vi "5800PRStatus.vi"(6 "VISA resource name":refnum<visa-resource-name>="GPIB::1") -> (9 "Gain":u16(ring) items=["20.0 dB", "40.0 dB", "60.0 dB"], 10 "Pan Scan Settings":T1, 11 "no 5800?":bool, 12 "Operation Mode":u16(ring) items=["Pulse-Echo", "Through", "External Pulser"], 13 "Output Attenuation":dbl=5.0 format="%.1g", 14 "Pulser Repitition Frequency":u16(ring)=10 items=["External Remote", "External BNC", "0.080 KHz", "0.100 KHz", "0.125 KHz", "0.160 KHz", "0.200 KHz", "0.250 KHz", "0.400 KHz", "0.500 KHz", "1.000 KHz", "1.250 KHz", "2.000 KHz", "2.500 KHz", "4.000 KHz", "5.000 KHz", "10.000 KHz"], 15 "Energy Level":u16(ring)=1 items=["12.5 uJ", "25.0 uJ", "50.0 uJ", "100.0 uJ"], 16 "Damping Value":u16(ring)=3 items=["15 ohms", "17 ohms", "21 ohms", "25 ohms", "36 ohms", "50 ohms", "100 ohms", "500 ohms"], 17 "Highpass Filter Frequency":u16(ring) items=["1 KHz", "100 KHz", "300 KHz", "1000 KHz"], 18 "Lowpass Filter Frequency":u16(ring)=3 items=["5 MHz", "10 MHz", "20 MHz", "35 MHz"], 19 "Input Attenuation":u16(ring)=1 items=["0.0 dB", "10.0 dB", "20.0 dB", "30.0 dB", "40.0 dB", "50.0 dB"])   [LabVIEW 2022 SP3]
panel:
  # "This VI returns the present setting of the 5800PR"
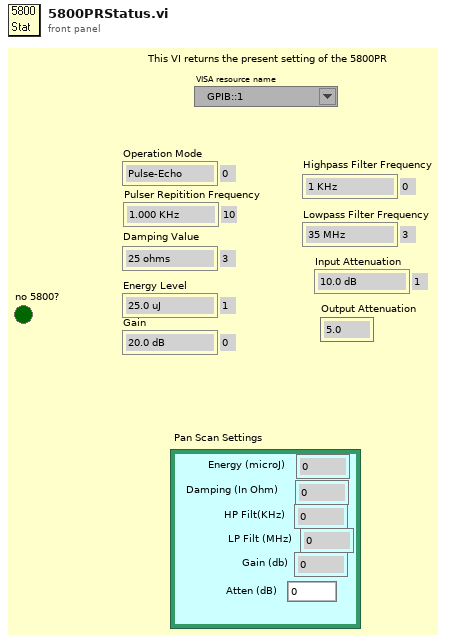
[diagram p1: front panel]
types:
  T1 = cluster{"Energy (microJ)":u8, "Damping (In Ohm)":u8, "HP Filt(KHz) ":u8, "LP Filt (MHz)":u8, "Gain (db)":u8, "Atten (dB)":sgl}
  T2 = cluster{"[0]":i32, "[1]":i32, "[2]":i32, "[3]":i32, "[4]":i32, "[5]":i32, "[6]":i32, "[7]":i32, "[8]":i32}
  T3 = cluster{"[5]":i32, "[2]":i32, "[1]":i32, "[0]":i32, "[3]":i32, i32}
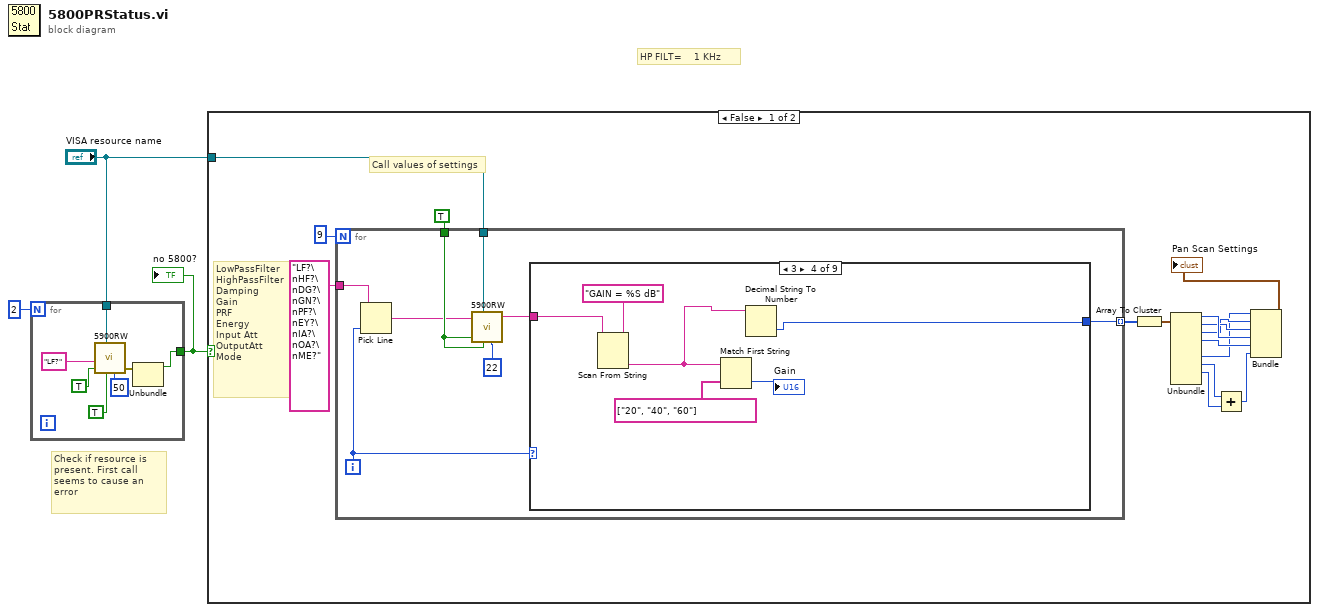
[diagram p0: block diagram]
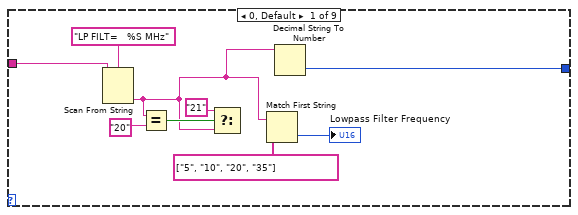
[diagram p2: hidden frame]
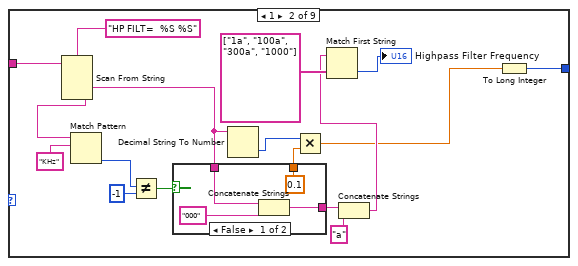
[diagram p3: hidden frame]
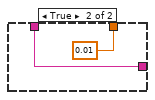
[diagram p4: hidden frame]
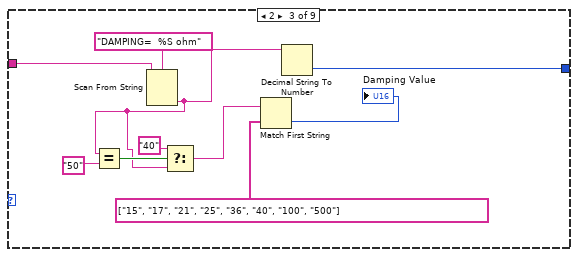
[diagram p5: hidden frame]
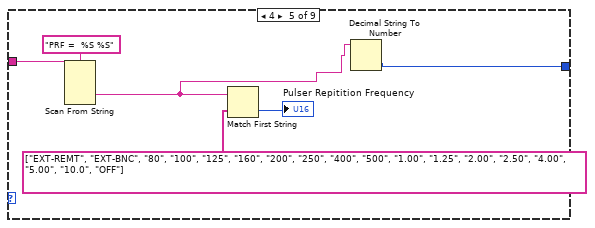
[diagram p6: hidden frame]
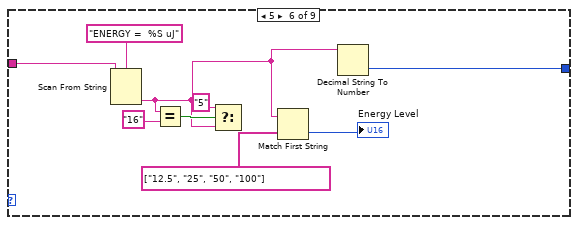
[diagram p7: hidden frame]
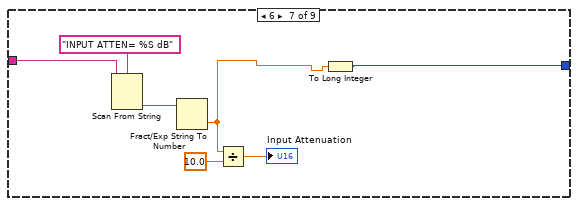
[diagram p8: hidden frame]
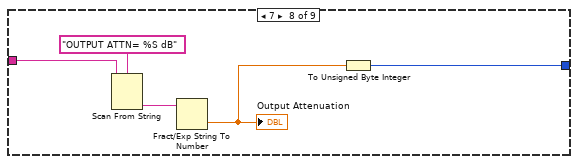
[diagram p9: hidden frame]
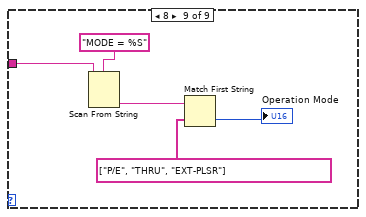
[diagram p10: hidden frame]
diagram:
  # "HP FILT=    1 KHz"
  # "Check if resource is present. First call seems to cause an error"
  n1 = for {
    N: 2 -> [_]
    tunnel: "VISA resource name" -> [w7]
    tunnel: [w5] -> w2
    n2 = call "5900RW.vi"("VISA resource name"=w7, "ENTER STRING"="LF?", "Read ?"=TRUE, "Write ?"=TRUE, "# bytes\nto read"=50) -> ("error out"=w6:errorcluster)  [unwired: 4 out]
    n3 = Unbundle(w6) -> ("status"=w5:bool)  [unwired: 2 out]
  }
  "no 5800?" <- w2
  n4 = case shown="False" w2 {
    tunnel: "VISA resource name" -> [w23 _]
    frame False {
      # "Call values of settings"
      # "LowPassFilter\nHighPassFilter\nDamping\nGain\nPRF\nEnergy\nInput Att\nOutputAtt\nMode"
      n5 = for {
        N: 9 -> [_]
        tunnel: TRUE -> [w33]
        tunnel: "LF?\nHF?\nDG?\nGN?\nPF?\nEY?\nIA?\nOA?\nME?" -> [w31]
        tunnel: w23 -> [w28]
        tunnel: [w26] -> w21 mode=indexing
        i -> [w30]
        n6 = Pick Line(multi-line string=w31, line index=w30) -> (output string=w32:string)  [unwired: 1 out]
        n7 = call "5900RW.vi"("VISA resource name"=w28, "ENTER STRING"=w32, "Read ?"=w33, "Write ?"=w33, "# bytes\nto read"=22) -> ("Characters Read"=w29:string)  [unwired: 1 in, 3 out]
        n8 = case shown="3" w30 {
          tunnel: w29 -> [w37 w51 w73 w79 w86 w91 w101 w106 w110]
          tunnel: [w34 w43 w66 w76 w82 w88 w97 w104 _] -> w26
          frame 0, Default {
            n9 = Scan From String(format string="LP FILT=   %S MHz", input string=w37) -> (output 1=w35:string)  [unwired: 2 in, 4 out]
            n10 = Equal?(x=w35, y="20") -> (x = y?=w40:bool)
            n11 = Select(t="21", s=w40, f=w35) -> ()  [unwired: 1 out]
            n12 = Match First String(2:string[] ["5", "10", "20", "35"], 3:w35) -> (0:→"Lowpass Filter Frequency":i32)  [unwired: 1 out]
            n13 = Decimal String To Number(string=w35) -> (number=w34:i32)  [unwired: 2 in, 1 out]
          }
          frame 1 {
            n14 = Scan From String(format string="HP FILT=  %S %S", input string=w51) -> (output 1=w47:string, output 2=w50:string)  [unwired: 2 in, 5 out]
            n15 = Match Pattern(string=w50, regular expression="KHz") -> (offset past match=w54:i32)  [unwired: 4 out]
            n16 = Not Equal?(x=w54, y=-1) -> (x != y?=w56:bool)
            n17 = case shown="False" w56 {
              tunnel: w47 -> [w61 w65]
              tunnel: [w62 w65] -> w58
              tunnel: [0.1 0.01] -> w45
              frame False {
                n18 = Concatenate Strings(w61, "000") -> (w62:string)
              }
              frame True {
              }
            }
            n19 = Decimal String To Number(string=w47) -> (number=w46:i32)  [unwired: 2 in, 1 out]
            n20 = Multiply(x=w46, y=w45) -> (x*y=w44:dbl)
            n21 = Concatenate Strings(w58, "a") -> (w49:string)
            n22 = Match First String(2:string[] ["1a", "100a", "300a", "1000"], 3:w49) -> (0:→"Highpass Filter Frequency":i32)  [unwired: 1 out]
            n23 = To Long Integer(number=w44) -> (32bit integer=w43:i32)
          }
          frame 2 {
            n24 = Scan From String(format string="DAMPING=  %S ohm", input string=w73) -> (output 1=w67:string)  [unwired: 2 in, 4 out]
            n25 = Equal?(x=w67, y="50") -> (x = y?=w71:bool)
            n26 = Select(t="40", s=w71, f=w67) -> (s? t:f=w68:string)
            n27 = Match First String(2:string[] ["15", "17", "21", "25", "36", "40", "100", "500"], 3:w68) -> (0:→"Damping Value":i32)  [unwired: 1 out]
            n28 = Decimal String To Number(string=w67) -> (number=w66:i32)  [unwired: 2 in, 1 out]
          }
          frame 3 {
            n29 = Scan From String(format string="GAIN = %S dB", input string=w79) -> (output 1=w77:string)  [unwired: 2 in, 4 out]
            n30 = Match First String(2:string[] ["20", "40", "60"], 3:w77) -> (0:→"Gain":i32)  [unwired: 1 out]
            n31 = Decimal String To Number(string=w77) -> (number=w76:i32)  [unwired: 2 in, 1 out]
          }
          frame 4 {
            n32 = Scan From String(format string="PRF =  %S %S", input string=w86) -> (output 1=w83:string)  [unwired: 2 in, 6 out]
            n33 = Match First String(2:string[] ["EXT-REMT", "EXT-BNC", "80", "100", "125", "160", "200", "250", "400", "500", "1.00", "1.25", "2.00", "2.50", "4.00", "5.00", "10.0", "OFF"], 3:w83) -> (0:→"Pulser Repitition Frequency":i32)  [unwired: 1 out]
            n34 = Decimal String To Number(string=w83) -> (number=w82:i32)  [unwired: 2 in, 1 out]
          }
          frame 5 {
            n35 = Scan From String(format string="ENERGY =  %S uJ", input string=w91) -> (output 1=w89:string)  [unwired: 2 in, 4 out]
            n36 = Equal?(x=w89, y="16") -> (x = y?=w94:bool)
            n37 = Select(t="5", s=w94, f=w89) -> ()  [unwired: 1 out]
            n38 = Match First String(2:string[] ["12.5", "25", "50", "100"], 3:w89) -> (0:→"Energy Level":i32)  [unwired: 1 out]
            n39 = Decimal String To Number(string=w89) -> (number=w88:i32)  [unwired: 2 in, 1 out]
          }
          frame 6 {
            n40 = Scan From String(format string="INPUT ATTEN= %S dB", input string=w101) -> (output 1=w103:string)  [unwired: 2 in, 4 out]
            n41 = Fract/Exp String To Number(string=w103) -> (number=w98:dbl)  [unwired: 4 out]
            n42 = Divide(x=w98, y=10.0) -> (x/y=→"Input Attenuation":dbl)
            n43 = To Long Integer(number=w98) -> (32bit integer=w97:i32)
          }
          frame 7 {
            n44 = Scan From String(format string="OUTPUT ATTN= %S dB", input string=w106) -> (output 1=w108:string)  [unwired: 2 in, 4 out]
            n45 = Fract/Exp String To Number(string=w108) -> (number=w105:dbl)  [unwired: 4 out]
            "Output Attenuation" <- w105
            n46 = To Unsigned Byte Integer(number=w105) -> (unsigned 8bit integer=w104:u8)
          }
          frame 8 {
            n47 = Scan From String(format string="MODE = %S", input string=w110) -> (output 1=w112:string)  [unwired: 2 in, 4 out]
            n48 = Match First String(2:string[] ["P/E", "THRU", "EXT-PLSR"], 3:w112) -> (0:→"Operation Mode":i32)  [unwired: 1 out]
          }
        }
      }
      n49 = Array To Cluster(array=w21) -> (cluster=w20:T2)
      n50 = Unbundle(w20) -> ("[0]"=w18:i32, "[1]"=w17:i32, "[2]"=w16:i32, "[3]"=w15:i32, "[5]"=w14:i32, "[6]"=w13:i32, "[7]"=w12:i32)  [unwired: 2 out]
      n51 = Add(x=w13, y=w12) -> (x+y=w11:i32)
      n52 = Bundle("[5]"=w14, "[2]"=w16, "[1]"=w17, "[0]"=w18, "[3]"=w15, w11) -> (→"Pan Scan Settings":T3)  [unwired: 1 in]
    }
    frame True {
    }
  }
